vi "SUB_Write_GeneralFile.vi"(1 "Filename":string, 2 "Text Input":string) -> (0 "err code":i32)   [LabVIEW 2011]
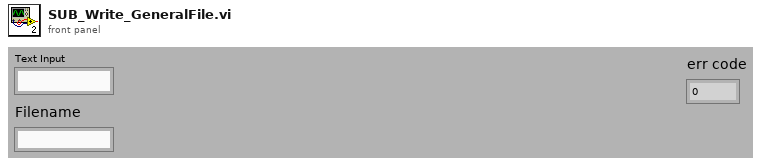
[diagram p1: front panel]
types:
  T1 = enum32{"invalid app kind", "Development System", "Run Time System", "Student Edition", "Embedded LabVIEW", "Evaluation", "Custom"}
  T2 = enum16{"open", "replace", "create", "open or create", "replace or create", "replace or create with confirmation"}
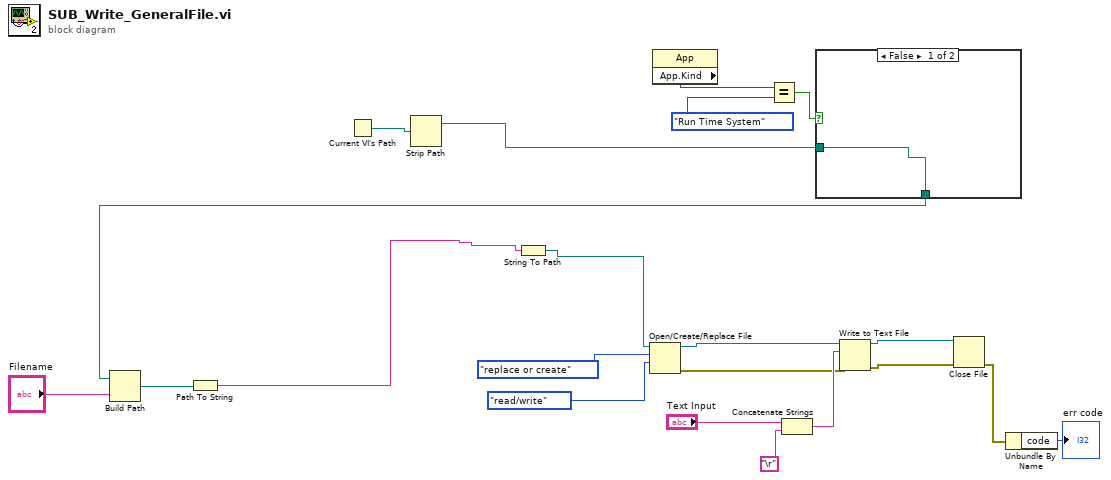
[diagram p0: block diagram]
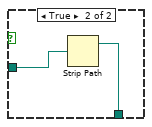
[diagram p2: hidden frame]
diagram:
  n1 = Current VI's Path() -> (path=w13:path)
  n2 = Strip Path(path=w13) -> (stripped path=w9:path)  [unwired: 1 out]
  n3 = property class="App"() -> ("App.Kind"=w12:T1)  [unwired: 2 in, 2 out]
  n4 = Equal?(x=w12, y=T1."Run Time System" ("Application:Kind")) -> (x = y?=w10:bool)
  n5 = Concatenate Strings("Text Input", "\r") -> (w18:string)
  n6 = case shown="False" w10 {
    tunnel: w9 -> [w22 w24]
    tunnel: [w22 w23] -> w5
    frame False {
    }
    frame True {
      n7 = Strip Path(path=w24) -> (stripped path=w23:path)  [unwired: 1 out]
    }
  }
  n8 = Build Path(base path=w5, name or relative path="Filename") -> (appended path=w6:path)
  n9 = Path To String(path=w6) -> (string=w4:string)
  n10 = String To Path(string=w4) -> (path=w8:path)
  n11 = Open/Create/Replace File(file path (use dialog)=w8, operation (0:open)=T2."replace or create", access (0:read/write)=enum16{"read/write", "read-only", "write-only"}."read/write") -> (refnum out=w17:refnum<file>, error out=w7:errorcluster)  [unwired: 3 in, 1 out]
  n12 = Write to Text File(file (use dialog)=w17, text=w18, error in=w7) -> (refnum out=w15:refnum<file>, error out=w16:errorcluster)  [unwired: 1 in, 1 out]
  n13 = Close File(refnum=w15, error in=w16) -> (error out=w2:errorcluster)  [unwired: 1 out]
  n14 = Unbundle By Name(w2) -> ("code"=→"err code":i32)
